vi "BattleShip.vi"() -> ()   [LabVIEW 2015]
uses:
  <vilib>/Utility/miscctls.llb/LVMouseTypeDef.ctl
  <vilib>/Utility/miscctls.llb/LVPoint32TypeDef.ctl
  <vilib>/Utility/miscctls.llb/LVPositionTypeDef.ctl
  <vilib>/picture/picture.llb/Draw True-Color Pixmap.vi
panel:
  out "appended path":path
  out "path":path
  out "BasePath":path
  in  "PlayMusic":i32
  out "HitIndex 4":u32
  out "HitIndex 3":u32
  out "Enum":T1(ring)
  out "TimeToChangeTurn":bool
  in  "First":bool
  in  "Counter":i32
  out "timed out 3":bool
  out "TimeToChangeTurn2 2":bool
  out "TimeToChangeTurn2":bool
  out "HitIndex 2":u32
  out "x .and. y? 4":bool
  out "x .and. y? 3":bool
  out "x .and. y? 2":bool
  out "x .and. y?":bool
  out "DataTemp":T2
  out "SendFormat":T2
  out "SendLocation":cluster{i32, i32}
  out "HitIndex":u32
  out "timed out 2":bool
  out "InputFromEnermy 2":T3
  out "timed out":bool
  out "InputFromEnermy":T3
  out "HitArray":picture[](array[picture])
  out "HitPicture":picture
  in  "MouseButtonDown":bool=TRUE
  out "Boolean":bool
  out "MouseLocation":T4
  out "Mouse Position":cluster{"X":i32, "Y":i32}
  in  "ClientFirst?":bool
  in  "URLReceive":string="dstp://localhost/dddd"
  in  "URLSend":string="dstp://localhost/wave"
  in  "BattleShipFace":bool[][](array[boolean])
  in  "BackGroundFace":bool[][](array[boolean])
  out "Mouse":T5
  out "InitArray":cluster{i32, i32}[](array[cluster])
  out "ShipFourArray":cluster{i32, i32}[][](array[cluster])
  out "ShipThreeArray":cluster{i32, i32}[][](array[cluster])
  out "ShipTwoArray":cluster{i32, i32}[][](array[cluster])
  out "ShipOneArray":cluster{i32, i32}[][](array[cluster])
  in  "ReadyButton":bool
  out "ShipMap":u32[][](array[numeric])
  out "ShipsNumber":i32[](array[numeric])
  in  "PictureButtonDown":bool
  out "ShipFourPixmap":u32[][](array[numeric]) format="%x"
  out "ShipThreePixmap":u32[][](array[numeric]) format="%x"
  out "ShipTwoPixmap":u32[][](array[numeric]) format="%x"
  out "ShipOnePixmap":u32[][](array[numeric]) format="%x"
  in  "Direction":i32
  out "PictureOut":picture
  in  "ShipChoose":i32
  out "BackGround":picture
  in  "ShipFour":bool
  in  "ShipThree":bool
  in  "ShipTwo":bool
  in  "ShipOne":bool
  in  "Array":bool[][](array[boolean])
  # "1.BattleShip的URLSend 要跟 BattleShip2的URLReceive 一樣\nBattleShip的 URLReceive 要跟 BattleShip2 的 URLSend 一樣\n，基本上用其中一個人的IP即可\nEX : BattleShip:\n            URLSend : dstp://140.113.89.154/wave \n            URLReceive : dstp://140.113.89.154/dddd\n         BattleShip2:\n            URLSend : dstp://140.113.89.154/dddd \n            URLReceive : dstp://140.113.89.154/wave\n\n\n2.一開始會先把船放到自己右邊的地圖上，然後每種船有固定的數量，按空白\n鍵可以轉船的方向，放完後，按Ready進入ReadyAndWait狀態，等BattleShip2\n的人也按Ready。如果連線成功，一方會進入MyTurn，另一邊會進入EnermyTurn\n，MyTurn的人可以用滑鼠按右邊地圖猜對面船的位子，如果猜中就可以繼續猜，\n沒中就要換邊，如果全部猜完，遊戲就會結束。\n\n3.連線後右邊是別人的地圖，左邊是自己的"
  # "遊戲狀態"
  # "Cruiser*4"
  # "Chaser*2"
  # "SubMarine*2"
  # "BattleShip*1"
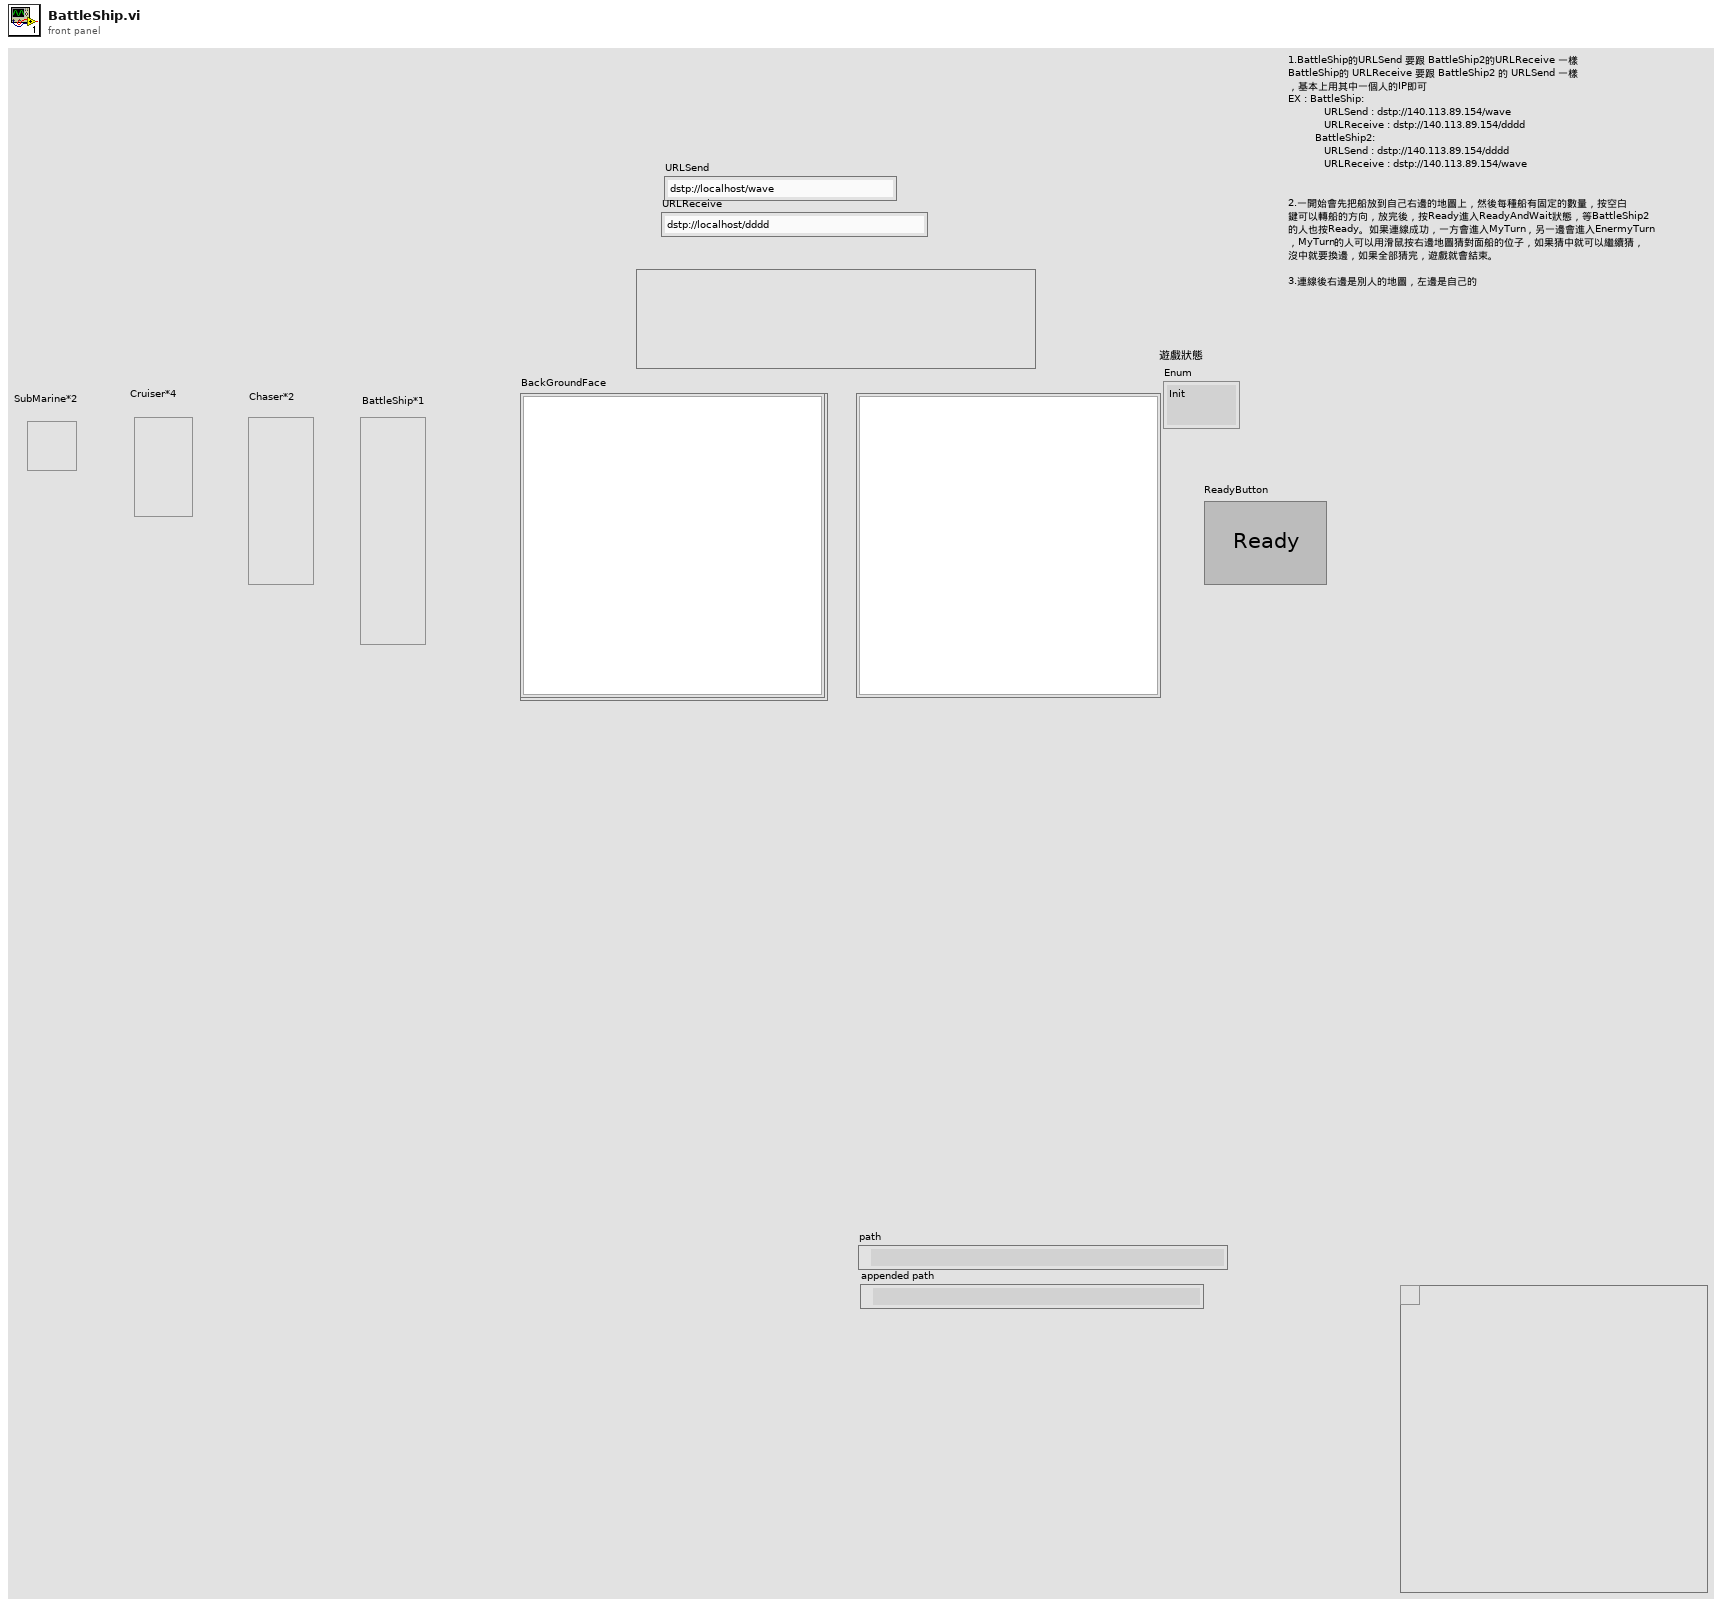
[diagram p1: front panel]
types:
  T1 = enum16{"Init", "Wait", "ReadyAndWait", "MyTurn", "EnermyTurn", "GameOver"}
  T2 = cluster{"HitIndex":u32, "SendLocation":cluster{i32, i32}}
  T3 = cluster{"BackGround":picture, "ShipMap":u32[][], "ShipOneArray":cluster{i32, i32}[][], "ShipTwoArray":cluster{i32, i32}[][], "ShipThreeArray":cluster{i32, i32}[][], "ShipFourArray":cluster{i32, i32}[][]}
  T4 = typedef "LVPoint32TypeDef.ctl" = cluster{"Horizontal":i32, "Vertical":i32}
  T5 = typedef "LVMouseTypeDef.ctl" = cluster{"Mouse Position":cluster{"X":i32, "Y":i32}, "Mouse Modifiers":cluster{"Button Down":bool, "Shift Mod":bool, "Menu Mod":bool, "Option Mod":bool}}
  T6 = enum16{"Init", "Wait", "ReadyAndWait", "MyTurn", "EnermyTurn"}
  T7 = cluster{"Button Down":bool, "Shift Mod":bool, "Menu Mod":bool, "Option Mod":bool}
  T8 = enum8{"Enabled", "Disabled", "Disabled and Grayed Out"}
  T9 = typedef "LVPositionTypeDef.ctl" = cluster{"Left":i32, "Top":i32}
  T10 = enum16{"Read", "Write", "ReadWrite", "BufferedRead", "BufferedReadWrite"}
  T11 = typedef "imagedata.ctl" = cluster{"image type":i32, "image depth":i32, "image":u8[], "mask":u8[], "colors":u32[], "Rectangle":cluster{"left":i16, "top":i16, "right":i16, "bottom":i16}}
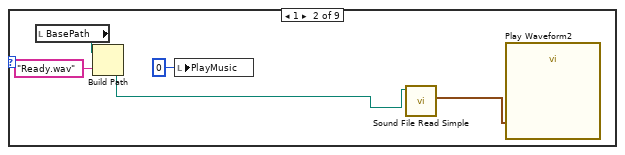
[diagram p3: hidden frame]
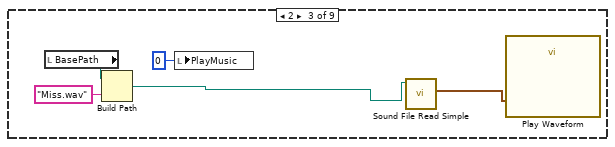
[diagram p4: hidden frame]
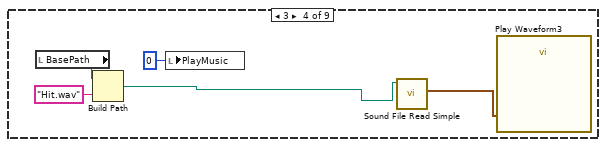
[diagram p5: hidden frame]
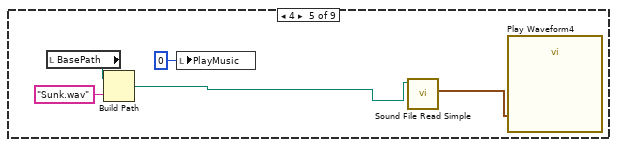
[diagram p6: hidden frame]
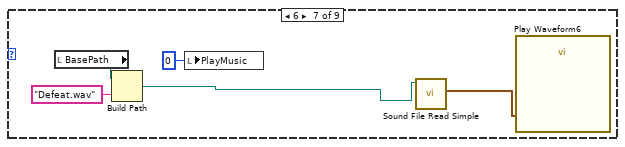
[diagram p7: hidden frame]
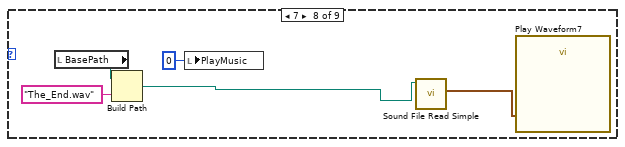
[diagram p8: hidden frame]
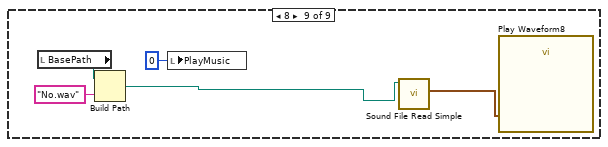
[diagram p9: hidden frame]
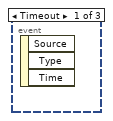
[diagram p10: hidden frame]
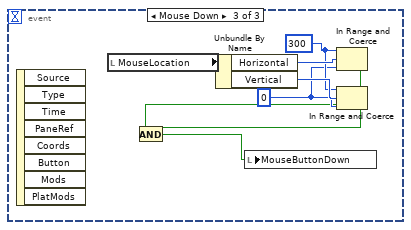
[diagram p11: hidden frame]
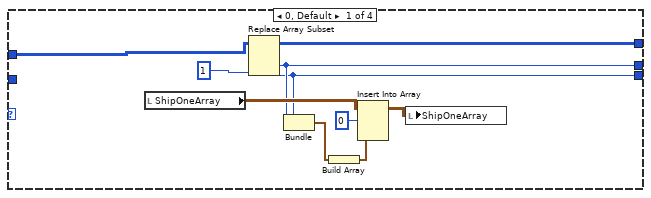
[diagram p13: hidden frame]
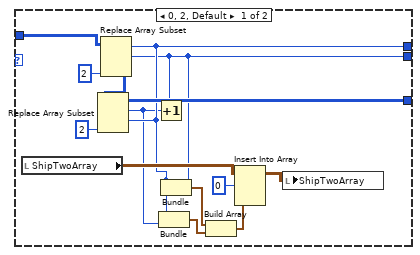
[diagram p14: hidden frame]
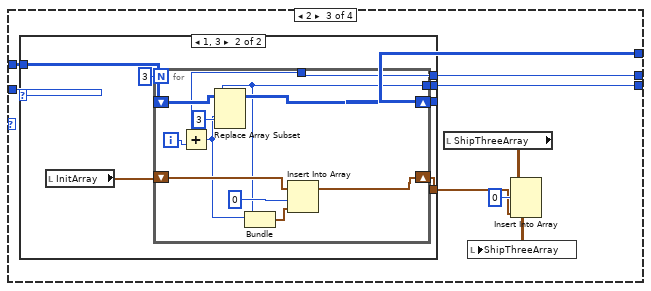
[diagram p15: hidden frame]
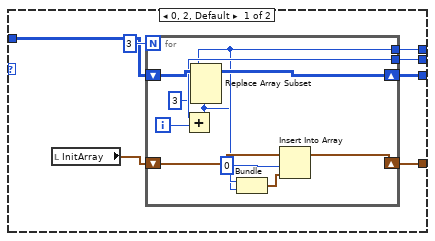
[diagram p16: hidden frame]
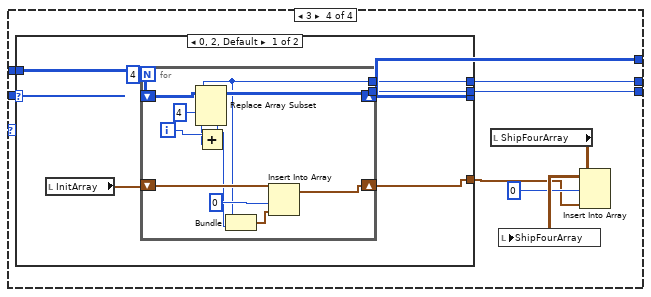
[diagram p17: hidden frame]
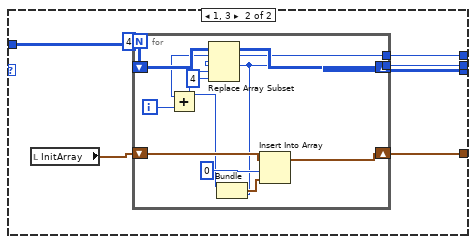
[diagram p18: hidden frame]
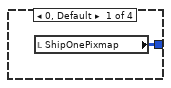
[diagram p19: hidden frame]
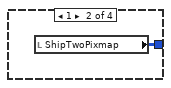
[diagram p20: hidden frame]
diagram:
  # "有五個State\n1.Init :\n           初始化必要的變數\n2.Wait:\n           畫製自己的地圖\n3.ReadyAndWait:\n           跟對方連線、傳資料\n4.MyTurn:\n           可以按右邊的地圖猜對方船的位子\n5.EnermyTurn:\n           對方的回合，被擊中的地方會畫上X\n6.GameOver:\n           遊戲結束"
  # "選定要放的音樂"
  # "在右邊的地圖上按滑鼠左鍵可以把選到的船印在圖上"
  # "把滑鼠移到右邊的地圖上時，會顯示應該會呈現的圖案"
  n1 = while {
    stop <- FALSE stop-if-true
    n2 = local read "Enum"() -> (w8:T1)
    n3 = Equal?(x=w8, y=T6."Wait") -> (x = y?=w7:bool)
    n4 = case shown="True" w7 {
      frame False {
      }
      frame True {
        w19 = 20 ("y")
        w25 = 20 ("y")
        n5 = local read "ShipChoose"() -> (w15:i32)
        n6 = case shown="3" w15 {
          tunnel: [w30 w31 w32 w33] -> w14
          frame 0, Default {
            n7 = local read "ShipOnePixmap"() -> (w30:u32[][])
          }
          frame 1 {
            n8 = local read "ShipTwoPixmap"() -> (w31:u32[][])
          }
          frame 2 {
            n9 = local read "ShipThreePixmap"() -> (w32:u32[][])
          }
          frame 3 {
            n10 = local read "ShipFourPixmap"() -> (w33:u32[][])
          }
        }
        n11 = property on="PictureOut" class="Pict"() -> ("Mouse"=w18:T5)  [unwired: 2 in, 2 out]
        n12 = local read "Direction"() -> (w17:i32)
        n13 = local read "BackGround"() -> (w28:picture)
        n14 = Unbundle By Name(w18) -> ("Mouse Position"=w29:cluster{"X":i32, "Y":i32}, "Mouse Modifiers"=w13:T7)
        "Mouse Position" <- w29
        n15 = case shown="3" w17 {
          tunnel: w14 -> [w34 w36 w40 w45]
          tunnel: [w34 w35 w37 w43] -> w16
          frame 0, Default {
          }
          frame 1 {
            n16 = Transpose 2D Array(2D array=w36) -> (transposed array=w35:u32[][])
          }
          frame 2 {
            n17 = Transpose 2D Array(2D array=w40) -> (transposed array=w39:u32[][])
            n18 = for {
              tunnel: w39 -> [w42] mode=indexing
              tunnel: [w41] -> w38 mode=indexing
              n19 = Reverse 1D Array(array=w42) -> (reversed array=w41:u32[])
            }
            n20 = Transpose 2D Array(2D array=w38) -> (transposed array=w37:u32[][])
          }
          frame 3 {
            n21 = Transpose 2D Array(2D array=w45) -> (transposed array=w44:u32[][])
            n22 = for {
              tunnel: w44 -> [w47] mode=indexing
              tunnel: [w46] -> w43 mode=indexing
              n23 = Reverse 1D Array(array=w47) -> (reversed array=w46:u32[])
            }
          }
        }
        n24 = Unbundle By Name(w13) -> ("Button Down"=w12:bool)
        n25 = Unbundle By Name(w29) -> ("X"=w27:i32, "Y"=w26:i32)
        n26 = Quotient & Remainder(x=w27, y=w25) -> (floor(x/y)=w21:i32)  [unwired: 1 out]
        n27 = Quotient & Remainder(x=w26, y=w25) -> (floor(x/y)=w22:i32)  [unwired: 1 out]
        n28 = local write "PictureButtonDown"(w12) -> ()
        n29 = Multiply(x=w21, y=w19) -> (x*y=w23:i32)
        n30 = Multiply(x=w19, y=w22) -> (x*y=w20:i32)
        n31 = Bundle(w23, w20) -> (w24:cluster{i32, i32})  [unwired: 1 in]
        n32 = call-poly <vilib>:"Draw Unflattened Pixmap.vi"("picture"=w28, "top left point(0, 0)"=w24, "data (RGB format)"=w16) -> ("new picture"=w11:picture)  [unwired: 6 in]
        n33 = local write "PictureOut"(w11) -> ()
      }
    }
  }
  n34 = while {
    stop <- FALSE stop-if-true
    n35 = local read "ShipsNumber"() -> (w52:i32[])
    n36 = local read "ShipChoose"() -> (w51:i32)
    n37 = local read "PictureButtonDown"() -> (w54:bool)
    n38 = Index Array(array=w52, index=w51) -> (element=w50:i32)
    n39 = Greater Than 0?(x=w50) -> (x > 0?=w49:bool)
    n40 = And(x=w54, y=w49) -> (x .and. y?=w53:bool)
    n41 = case shown="True" w53 {
      frame False {
      }
      frame True {
        w77 = 20 ("y")
        w73 = 20 ("y")
        n42 = local read "ShipsNumber"() -> (w63:i32[])
        n43 = local read "ShipChoose"() -> (w61:i32)
        n44 = case shown="3" w61 {
          tunnel: [w212 w213 w214 w215] -> w79
          frame 0, Default {
            n45 = local read "ShipOnePixmap"() -> (w212:u32[][])
          }
          frame 1 {
            n46 = local read "ShipTwoPixmap"() -> (w213:u32[][])
          }
          frame 2 {
            n47 = local read "ShipThreePixmap"() -> (w214:u32[][])
          }
          frame 3 {
            n48 = local read "ShipFourPixmap"() -> (w215:u32[][])
          }
        }
        n49 = property on="PictureOut" class="Pict"() -> ("Mouse"=w68:T5)  [unwired: 2 in, 2 out]
        n50 = local read "ShipMap"() -> (w60:u32[][])
        n51 = local read "Direction"() -> (w56:i32)
        n52 = Index Array(array=w63, index=w61) -> (element=w64:i32)
        n53 = Decrement(x=w64) -> (x-1=w66:i32)
        n54 = local read "BackGround"() -> (w70:picture)
        n55 = Replace Array Subset(array=w63, new element=w66, index=w61) -> (w65:i32[])
        n56 = Unbundle By Name(w68) -> ("Mouse Position"=w69:cluster{"X":i32, "Y":i32})
        n57 = case shown="3" w56 {
          tunnel: w79 -> [w216 w218 w222 w227]
          tunnel: [w216 w217 w219 w225] -> w78
          frame 0, Default {
          }
          frame 1 {
            n58 = Transpose 2D Array(2D array=w218) -> (transposed array=w217:u32[][])
          }
          frame 2 {
            n59 = Transpose 2D Array(2D array=w222) -> (transposed array=w221:u32[][])
            n60 = for {
              tunnel: w221 -> [w224] mode=indexing
              tunnel: [w223] -> w220 mode=indexing
              n61 = Reverse 1D Array(array=w224) -> (reversed array=w223:u32[])
            }
            n62 = Transpose 2D Array(2D array=w220) -> (transposed array=w219:u32[][])
          }
          frame 3 {
            n63 = Transpose 2D Array(2D array=w227) -> (transposed array=w226:u32[][])
            n64 = for {
              tunnel: w226 -> [w229] mode=indexing
              tunnel: [w228] -> w225 mode=indexing
              n65 = Reverse 1D Array(array=w229) -> (reversed array=w228:u32[])
            }
          }
        }
        n66 = local write "ShipsNumber"(w65) -> ()
        n67 = Unbundle By Name(w69) -> ("X"=w71:i32, "Y"=w72:i32)
        n68 = Quotient & Remainder(x=w71, y=w73) -> (floor(x/y)=w59:i32)  [unwired: 1 out]
        n69 = Quotient & Remainder(x=w72, y=w73) -> (floor(x/y)=w58:i32)  [unwired: 1 out]
        n70 = case shown="1" w61 {
          tunnel: w60 -> [w89 w93 w129 w174]
          tunnel: w59 -> [w84 w91 w127 w171]
          tunnel: w58 -> [w83 w92 w128 w172]
          tunnel: [w87 w90 w126 w173] -> w57
          tunnel: w56 -> [_ w94 w130 w175]
          frame 0, Default {
            n71 = local read "ShipOneArray"() -> (w85:cluster{i32, i32}[][])
            n72 = Replace Array Subset(array=w89, new element=u32 1 ("new element/subarray"), index (row)=w83, index (col)=w84) -> (w87:u32[][])
            n73 = Bundle(w84, w83) -> (w82:cluster{i32, i32})  [unwired: 1 in]
            n74 = Build Array(w82) -> (w81:cluster{i32, i32}[])
            n75 = Insert Into Array(array=w85, index (row)=0 ("index"), new element=w81) -> (w80:cluster{i32, i32}[][])  [unwired: 1 in]
            n76 = local write "ShipOneArray"(w80) -> ()
          }
          frame 1 {
            n77 = case shown="1, 3" w94 {
              tunnel: w93 -> [w108 w121]
              tunnel: w92 -> [w96 w109]
              tunnel: w91 -> [w97 w110]
              tunnel: [w104 w118] -> w90
              frame 0, 2, Default {
                n78 = local read "ShipTwoArray"() -> (w102:cluster{i32, i32}[][])
                n79 = Replace Array Subset(array=w108, new element=u32 2 ("new element/subarray"), index (row)=w96, index (col)=w97) -> (w105:u32[][])
                n80 = Increment(x=w96) -> (x+1=w95:i32)
                n81 = Replace Array Subset(array=w105, new element=u32 2 ("new element/subarray"), index (row)=w95, index (col)=w97) -> (w104:u32[][])
                n82 = Bundle(w97, w95) -> (w98:cluster{i32, i32})  [unwired: 1 in]
                n83 = Bundle(w97, w96) -> (w101:cluster{i32, i32})  [unwired: 1 in]
                n84 = Build Array(w101, w98) -> (w100:cluster{i32, i32}[])
                n85 = Insert Into Array(array=w102, index (row)=0 ("index"), new element=w100) -> (w99:cluster{i32, i32}[][])  [unwired: 1 in]
                n86 = local write "ShipTwoArray"(w99) -> ()
              }
              frame 1, 3 {
                w119 = u32 2 ("new element/subarray")
                n87 = local read "ShipTwoArray"() -> (w116:cluster{i32, i32}[][])
                n88 = Replace Array Subset(array=w121, new element=w119, index (row)=w109, index (col)=w110) -> (w120:u32[][])
                n89 = Increment(x=w110) -> (x+1=w111:i32)
                n90 = Replace Array Subset(array=w120, new element=w119, index (row)=w109, index (col)=w111) -> (w118:u32[][])
                n91 = Bundle(w111, w109) -> (w112:cluster{i32, i32})  [unwired: 1 in]
                n92 = Bundle(w110, w109) -> (w115:cluster{i32, i32})  [unwired: 1 in]
                n93 = Build Array(w115, w112) -> (w114:cluster{i32, i32}[])
                n94 = Insert Into Array(array=w116, index (row)=0 ("index"), new element=w114) -> (w113:cluster{i32, i32}[][])  [unwired: 1 in]
                n95 = local write "ShipTwoArray"(w113) -> ()
              }
            }
          }
          frame 2 {
            n96 = case shown="1, 3" w130 {
              tunnel: w129 -> [w136 w154]
              tunnel: w128 -> [w135 w152]
              tunnel: w127 -> [w134 w153]
              tunnel: [w133 w151] -> w126
              tunnel: [w131 w149] -> w123
              frame 0, 2, Default {
                n97 = local read "InitArray"() -> (w132:cluster{i32, i32}[])
                n98 = for {
                  N: 3 -> [_]
                  shift-right: [w147] -> w133
                  shift-left: w136 -> [w148]
                  tunnel: w135 -> [w145]
                  tunnel: w134 -> [w141]
                  shift-right: [w138] -> w131
                  shift-left: w132 -> [w143]
                  i -> [w146]
                  n99 = Add(x=w145, y=w146) -> (x+y=w140:i32)
                  n100 = Replace Array Subset(array=w148, new element=u32 3 ("new element/subarray"), index (row)=w140, index (col)=w141) -> (w147:u32[][])
                  n101 = Bundle(w141, w140) -> (w139:cluster{i32, i32})  [unwired: 1 in]
                  n102 = Insert Into Array(array=w143, index=0, new element=w139) -> (w138:cluster{i32, i32}[])
                }
              }
              frame 1, 3 {
                n103 = local read "InitArray"() -> (w150:cluster{i32, i32}[])
                n104 = for {
                  N: 3 -> [_]
                  shift-right: [w165] -> w151
                  shift-left: w154 -> [w166]
                  tunnel: w153 -> [w163]
                  tunnel: w152 -> [w156]
                  shift-right: [w158] -> w149
                  shift-left: w150 -> [w159]
                  i -> [w164]
                  n105 = Add(x=w163, y=w164) -> (x+y=w157:i32)
                  n106 = Replace Array Subset(array=w166, new element=u32 3 ("new element/subarray"), index (row)=w156, index (col)=w157) -> (w165:u32[][])
                  n107 = Bundle(w157, w156) -> (w160:cluster{i32, i32})  [unwired: 1 in]
                  n108 = Insert Into Array(array=w159, index=0, new element=w160) -> (w158:cluster{i32, i32}[])
                }
              }
            }
            n109 = local read "ShipThreeArray"() -> (w125:cluster{i32, i32}[][])
            n110 = Insert Into Array(array=w125, index (row)=0, new element=w123) -> (w122:cluster{i32, i32}[][])  [unwired: 1 in]
            n111 = local write "ShipThreeArray"(w122) -> ()
          }
          frame 3 {
            n112 = case shown="0, 2, Default" w175 {
              tunnel: w174 -> [w182 w199]
              tunnel: [w181 w196] -> w173
              tunnel: w172 -> [w179 w197]
              tunnel: w171 -> [w178 w198]
              tunnel: [w176 w194] -> w167
              frame 0, 2, Default {
                n113 = local read "InitArray"() -> (w177:cluster{i32, i32}[])
                n114 = for {
                  N: 4 -> [_]
                  shift-right: [w192] -> w181
                  shift-left: w182 -> [w193]
                  tunnel: w179 -> [w190]
                  tunnel: w178 -> [w183]
                  shift-right: [w185] -> w176
                  shift-left: w177 -> [w186]
                  i -> [w191]
                  n115 = Add(x=w191, y=w190) -> (x+y=w184:i32)
                  n116 = Replace Array Subset(array=w193, new element=u32 4 ("new element/subarray"), index (row)=w184, index (col)=w183) -> (w192:u32[][])
                  n117 = Bundle(w183, w184) -> (w187:cluster{i32, i32})  [unwired: 1 in]
                  n118 = Insert Into Array(array=w186, index=0, new element=w187) -> (w185:cluster{i32, i32}[])
                }
              }
              frame 1, 3 {
                n119 = local read "InitArray"() -> (w195:cluster{i32, i32}[])
                n120 = for {
                  N: 4 -> [_]
                  shift-right: [w210] -> w196
                  shift-left: w199 -> [w211]
                  tunnel: w198 -> [w203]
                  tunnel: w197 -> [w201]
                  shift-right: [w204] -> w194
                  shift-left: w195 -> [w205]
                  i -> [w209]
                  n121 = Add(x=w203, y=w209) -> (x+y=w202:i32)
                  n122 = Replace Array Subset(array=w211, new element=u32 4 ("new element/subarray"), index (row)=w201, index (col)=w202) -> (w210:u32[][])
                  n123 = Bundle(w202, w201) -> (w206:cluster{i32, i32})  [unwired: 1 in]
                  n124 = Insert Into Array(array=w205, index=0, new element=w206) -> (w204:cluster{i32, i32}[])
                }
              }
            }
            n125 = local read "ShipFourArray"() -> (w169:cluster{i32, i32}[][])
            n126 = Insert Into Array(array=w169, index (row)=0 ("index"), new element=w167) -> (w170:cluster{i32, i32}[][])  [unwired: 1 in]
            n127 = local write "ShipFourArray"(w170) -> ()
          }
        }
        n128 = Multiply(x=w59, y=w77) -> (x*y=w75:i32)
        n129 = Multiply(x=w77, y=w58) -> (x*y=w76:i32)
        n130 = Bundle(w75, w76) -> (w74:cluster{i32, i32})  [unwired: 1 in]
        n131 = call-poly <vilib>:"Draw Unflattened Pixmap.vi"("picture"=w70, "top left point(0, 0)"=w74, "data (RGB format)"=w78) -> ("new picture"=w67:picture)  [unwired: 6 in]
        n132 = local write "ShipMap"(w57) -> ()
        n133 = local write "BackGround"(w67) -> ()
        n134 = Wait Until Next ms Multiple(millisecond multiple=u32 1500) -> ()  [unwired: 1 out]
      }
    }
    n135 = property on="PictureOut" class="Pict"() -> ("Mouse"=→"Mouse":T5)  [unwired: 2 in, 2 out]
  }
  n136 = while {
    shift-right: [w231] -> _
    shift-left: T1."Init" -> [w230]
    stop <- FALSE stop-if-true
    n137 = case shown="\"Wait\"" w230 {
      tunnel: [enum16{"Init", "Wait"}."Wait" enum16{"Init", "Wait"}."Wait" w345 w391 w510 w751 T1."GameOver"] -> w231
      frame "Init" {
        w285 = FALSE
        w300 = 15
        w303 = 15
        n138 = local write "ShipChoose"(0 ("ShipChoose")) -> ()
        n139 = Initialize Array(cluster{i32, i32} {0, 0}, 0 ("dimension size"), 0 ("dimension size")) -> (→"ShipOneArray" →"ShipTwoArray" →"ShipThreeArray" →"ShipFourArray":cluster{i32, i32}[][])
        n140 = local write "PlayMusic"(0 ("PlayMusic")) -> ()
        n141 = local write "Direction"(0 ("Direction")) -> ()
        n142 = Initialize Array(u32 0 ("element"), 15 ("dimension size"), 15 ("dimension size")) -> (→"ShipMap":u32[][])
        n143 = Build Array(2, 4, 2, 1) -> (→"ShipsNumber":i32[])
        n144 = local read "BasePath"() -> (w276:path)
        n145 = local read "BasePath"() -> (w272:path)
        n146 = Build Path(base path=w276, name or relative path="ShipTwo.png") -> (appended path=w277:path)
        n147 = call <vilib>:"Read PNG File.vi"("path to PNG file"=w277) -> ("image data"=w341:T11)  [unwired: 8 in, 2 out]
        n148 = call <vilib>:"Unflatten Pixmap.vi"("image data"=w341) -> ("24-bit pixmap"=→"ShipTwoPixmap":u32[][])  [unwired: 4 in, 6 out]
        n149 = Build Path(base path=w276, name or relative path="BackGroundWhite.png") -> (appended path=w281:path)
        n150 = call <vilib>:"Read PNG File.vi"("path to PNG file"=w281) -> ("image data"=w337:T11)  [unwired: 8 in, 2 out]
        n151 = call <vilib>:"Unflatten Pixmap.vi"("image data"=w337) -> ("24-bit pixmap"=w336:u32[][])  [unwired: 4 in, 6 out]
        n152 = call-poly <vilib>:"Draw Unflattened Pixmap.vi"("data (RGB format)"=w336) -> ("new picture"=w335:picture)  [unwired: 8 in]
        n153 = local write "BackGround"(w335) -> ()
        n154 = Build Path(base path=w272, name or relative path="ShipThree.png") -> (appended path=w271:path)
        n155 = call <vilib>:"Read PNG File.vi"("path to PNG file"=w271) -> ("image data"=w340:T11)  [unwired: 8 in, 2 out]
        n156 = call <vilib>:"Unflatten Pixmap.vi"("image data"=w340) -> ("24-bit pixmap"=→"ShipThreePixmap":u32[][])  [unwired: 4 in, 6 out]
        n157 = Build Path(base path=w276, name or relative path="ShipOne.png") -> (appended path=w278:path)
        n158 = call <vilib>:"Read PNG File.vi"("path to PNG file"=w278) -> ("image data"=w342:T11)  [unwired: 8 in, 2 out]
        n159 = call <vilib>:"Unflatten Pixmap.vi"("image data"=w342) -> ("24-bit pixmap"=→"ShipOnePixmap":u32[][])  [unwired: 4 in, 6 out]
        n160 = Build Path(base path=w272, name or relative path="ShipFour.png") -> (appended path=w270:path)
        n161 = call <vilib>:"Read PNG File.vi"("path to PNG file"=w270) -> ("image data"=w339:T11)  [unwired: 8 in, 2 out]
        n162 = call <vilib>:"Unflatten Pixmap.vi"("image data"=w339) -> ("24-bit pixmap"=→"ShipFourPixmap":u32[][])  [unwired: 4 in, 6 out]
        n163 = local read "BasePath"() -> (w260:path)
        n164 = local read "BasePath"() -> (w263:path)
        n165 = local read "BasePath"() -> (w268:path)
        n166 = local read "BasePath"() -> (w267:path)
        n167 = local read "BasePath"() -> (w264:path)
        n168 = Build Path(base path=w260, name or relative path="HitBattleship.png") -> (appended path=w255:path)
        n169 = Build Path(base path=w263, name or relative path="HitChaser.png") -> (appended path=w256:path)
        n170 = Build Path(base path=w268, name or relative path="TextBackGround.png") -> (appended path=w259:path)
        n171 = Build Path(base path=w267, name or relative path="HitSubMarine.png") -> (appended path=w258:path)
        n172 = Build Path(base path=w264, name or relative path="HitCruiser.png") -> (appended path=w257:path)
        n173 = property on="BackGroundFace" class="Arr (strict)"("DisabledEnum"=T8."Disabled" ("Disabled")) -> ()  [unwired: 2 in, 2 out]
        n174 = local write "ClientFirst?"(TRUE ("ClientFirst?")) -> ()
        n175 = local write "HitIndex 2"(u32 0 ("HitIndex 2")) -> ()
        n176 = local write "HitIndex"(u32 0 ("HitIndex 2")) -> ()
        n177 = local read "BasePath"() -> (w244:path)
        n178 = local read "BasePath"() -> (w245:path)
        n179 = local read "BasePath"() -> (w253:path)
        n180 = local read "BasePath"() -> (w252:path)
        n181 = local read "BasePath"() -> (w248:path)
        n182 = local read "BasePath"() -> (w249:path)
        n183 = Build Path(base path=w244, name or relative path="SunkBattleShip.png") -> (appended path=w239:path)
        n184 = Build Path(base path=w245, name or relative path="Win.png") -> (appended path=w238:path)
        n185 = Build Path(base path=w253, name or relative path="SunkSubmarine.png") -> (appended path=w242:path)
        n186 = Build Path(base path=w252, name or relative path="SunkCruiser.png") -> (appended path=w241:path)
        n187 = Build Path(base path=w248, name or relative path="Lose.png") -> (appended path=w237:path)
        "appended path" <- w237
        n188 = Build Path(base path=w249, name or relative path="SunkChaser.png") -> (appended path=w240:path)
        n189 = Initialize Array(FALSE, w303, w303) -> (w298:bool[][])
        n190 = Initialize Array(FALSE, w300, w300) -> (w299:bool[][])
        n191 = local write "BattleShipFace"(w299) -> ()
        n192 = local write "BackGroundFace"(w298) -> ()
        n193 = property on="BattleShipFace" class="Arr (strict)"("Position"=T9 {"Left"=1000, "Top"=1000}) -> ()  [unwired: 2 in, 2 out]
        n194 = local write "MouseButtonDown"(FALSE ("MouseButtonDown")) -> ()
        n195 = local write "TimeToChangeTurn"(w285) -> ()
        n196 = local write "TimeToChangeTurn2"(w285) -> ()
        n197 = property on="Boolean" class="Bool (strict)"("Position"=T9 {"Left"=1000, "Top"=1000}) -> ()  [unwired: 2 in, 2 out]
        n198 = call <vilib>:"Read PNG File.vi"("path to PNG file"=w237) -> ("image data"=w289:T11)  [unwired: 8 in, 2 out]
        n199 = call <vilib>:"Read PNG File.vi"("path to PNG file"=w238) -> ("image data"=w288:T11)  [unwired: 8 in, 2 out]
        n200 = call <vilib>:"Read PNG File.vi"("path to PNG file"=w255) -> ("image data"=w311:T11)  [unwired: 8 in, 2 out]
        n201 = call <vilib>:"Read PNG File.vi"("path to PNG file"=w241) -> ("image data"=w296:T11)  [unwired: 8 in, 2 out]
        n202 = call <vilib>:"Read PNG File.vi"("path to PNG file"=w258) -> ("image data"=w314:T11)  [unwired: 8 in, 2 out]
        n203 = call <vilib>:"Read PNG File.vi"("path to PNG file"=w239) -> ("image data"=w294:T11)  [unwired: 8 in, 2 out]
        n204 = call <vilib>:"Read PNG File.vi"("path to PNG file"=w242) -> ("image data"=w297:T11)  [unwired: 8 in, 2 out]
        n205 = call <vilib>:"Read PNG File.vi"("path to PNG file"=w240) -> ("image data"=w295:T11)  [unwired: 8 in, 2 out]
        n206 = call <vilib>:"Read PNG File.vi"("path to PNG file"=w257) -> ("image data"=w313:T11)  [unwired: 8 in, 2 out]
        n207 = call <vilib>:"Read PNG File.vi"("path to PNG file"=w256) -> ("image data"=w312:T11)  [unwired: 8 in, 2 out]
        n208 = call <vilib>:"Read PNG File.vi"("path to PNG file"=w259) -> ("image data"=w310:T11)  [unwired: 8 in, 2 out]
        n209 = call <vilib>:"Draw Flattened Pixmap.vi"("image data"=w289) -> ("new picture"=w286:picture)  [unwired: 8 in]
        n210 = call <vilib>:"Draw Flattened Pixmap.vi"("image data"=w288) -> ("new picture"=w287:picture)  [unwired: 8 in]
        n211 = call <vilib>:"Draw Flattened Pixmap.vi"("image data"=w311) -> ("new picture"=w305:picture)  [unwired: 8 in]
        n212 = call <vilib>:"Draw Flattened Pixmap.vi"("image data"=w296) -> ("new picture"=w292:picture)  [unwired: 8 in]
        n213 = call <vilib>:"Draw Flattened Pixmap.vi"("image data"=w314) -> ("new picture"=w308:picture)  [unwired: 8 in]
        n214 = call <vilib>:"Draw Flattened Pixmap.vi"("image data"=w294) -> ("new picture"=w290:picture)  [unwired: 8 in]
        n215 = call <vilib>:"Draw Flattened Pixmap.vi"("image data"=w297) -> ("new picture"=w293:picture)  [unwired: 8 in]
        n216 = call <vilib>:"Draw Flattened Pixmap.vi"("image data"=w295) -> ("new picture"=w291:picture)  [unwired: 8 in]
        n217 = call <vilib>:"Draw Flattened Pixmap.vi"("image data"=w313) -> ("new picture"=w307:picture)  [unwired: 8 in]
        n218 = call <vilib>:"Draw Flattened Pixmap.vi"("image data"=w312) -> ("new picture"=w306:picture)  [unwired: 8 in]
        n219 = call <vilib>:"Draw Flattened Pixmap.vi"("image data"=w310) -> ("new picture"=w309:picture)  [unwired: 8 in]
        n220 = local write "First"(TRUE ("First")) -> ()
        n221 = Build Array(w309, w308, w307, w306, w305, w293, w292, w291, w290, w287, w286) -> (→"HitArray":picture[])
      }
      frame Default {
      }
      frame "Wait" {
        n222 = event shown="[6] \"ReadyButton\": Mouse Down" {
          selector: _ -> [_ _ _ _ _ _ _]
          dyn-events: _ -> [_ _ _ _ _ _ _]
          timeout: _ -> [_ _ _ _ _ _ _]
          tunnel: [_ enum16{"Init", "Wait", "ReadyAndWait"}."Wait" enum16{"Init", "Wait", "ReadyAndWait"}."Wait" enum16{"Init", "Wait", "ReadyAndWait"}."Wait" enum16{"Init", "Wait", "ReadyAndWait"}."Wait" enum16{"Init", "Wait", "ReadyAndWait"}."Wait" w381] -> w345
          event Timeout {
            n223 = event-data() -> ()  [unwired: 1 in, 3 out]
          }
          event "ShipOne": Mouse Down {
            w349 = 0 ("ShipChoose")
            n224 = event-data() -> ()  [unwired: 1 in, 8 out]
            n225 = local read "ShipsNumber"() -> (w352:i32[])
            n226 = Index Array(array=w352, index=w349) -> (element=w351:i32)
            n227 = local read "ShipChoose"() -> (w347:i32)
            n228 = Greater Than 0?(x=w351) -> (x > 0?=w350:bool)
            n229 = Select(t=w349, s=w350, f=w347) -> (s? t:f=w348:i32)
            n230 = local write "ShipChoose"(w348) -> ()
          }
          event "ShipTwo": Mouse Down {
            w356 = 1 ("ShipChoose")
            n231 = event-data() -> ()  [unwired: 1 in, 8 out]
            n232 = local read "ShipsNumber"() -> (w359:i32[])
            n233 = Index Array(array=w359, index=w356) -> (element=w358:i32)
            n234 = local read "ShipChoose"() -> (w354:i32)
            n235 = Greater Than 0?(x=w358) -> (x > 0?=w357:bool)
            n236 = Select(t=w356, s=w357, f=w354) -> (s? t:f=w355:i32)
            n237 = local write "ShipChoose"(w355) -> ()
          }
          event "ShipThree": Mouse Down {
            w365 = 2 ("ShipChoose")
            n238 = event-data() -> ()  [unwired: 1 in, 8 out]
            n239 = local read "ShipsNumber"() -> (w364:i32[])
            n240 = Index Array(array=w364, index=w365) -> (element=w363:i32)
            n241 = local read "ShipChoose"() -> (w366:i32)
            n242 = Greater Than 0?(x=w363) -> (x > 0?=w362:bool)
            n243 = Select(t=w365, s=w362, f=w366) -> (s? t:f=w361:i32)
            n244 = local write "ShipChoose"(w361) -> ()
          }
          event "ShipFour": Mouse Down {
            w370 = 3 ("ShipChoose")
            n245 = event-data() -> ()  [unwired: 1 in, 8 out]
            n246 = local read "ShipsNumber"() -> (w373:i32[])
            n247 = Index Array(array=w373, index=w370) -> (element=w372:i32)
            n248 = local read "ShipChoose"() -> (w368:i32)
            n249 = Greater Than 0?(x=w372) -> (x > 0?=w371:bool)
            n250 = Select(t=w370, s=w371, f=w368) -> (s? t:f=w369:i32)
            n251 = local write "ShipChoose"(w369) -> ()
          }
          event Key Down {
            n252 = event-data() -> ("ScanCode"=w375:i16)  [unwired: 1 in, 9 out]
            n253 = case shown="57" w375 {
              frame 0, Default {
              }
              frame 57 {
                n254 = local read "Direction"() -> (w379:i32)
                n255 = Increment(x=w379) -> (x+1=w378:i32)
                n256 = Quotient & Remainder(x=w378, y=4) -> (x-y*floor(x/y)=w376:i32)  [unwired: 1 out]
                n257 = local write "Direction"(w376) -> ()
              }
            }
          }
          event "ReadyButton": Mouse Down {
            n258 = event-data() -> ()  [unwired: 1 in, 8 out]
            n259 = local read "ShipsNumber"() -> (w385:i32[])
            n260 = for {
              shift-right: [w387] -> w384
              shift-left: TRUE -> [w388]
              tunnel: w385 -> [w390] mode=indexing
              n261 = Equal To 0?(x=w390) -> (x = 0?=w389:bool)
              n262 = And(x=w389, y=w388) -> (x .and. y?=w387:bool)
            }
            n263 = local write "PlayMusic"(1 ("PlayMusic")) -> ()
            n264 = Select(t=enum16{"Init", "Wait", "ReadyAndWait"}."ReadyAndWait", s=w384, f=enum16{"Init", "Wait", "ReadyAndWait"}."ReadyAndWait") -> (s? t:f=w381:enum16{"Init", "Wait", "ReadyAndWait"})
          }
        }
      }
      frame "ReadyAndWait" {
        n265 = flat-sequence {
          frame #0 {
            n266 = property on="PictureOut" class="Pict"() -> ("Position"=w399:T9)  [unwired: 2 in, 2 out]
            n267 = Unbundle By Name(w399) -> ("Left"=w400:i32, "Top"=w396:i32)
            n268 = Decrement(x=w400) -> (x-1=w397:i32)
            n269 = Decrement(x=w396) -> (x-1=w395:i32)
            n270 = Bundle(cluster=w399, "Left"=w397, "Top"=w395) -> (w398:T9)
            n271 = property on="BattleShipFace" class="Arr (strict)"("Position"=w398) -> ()  [unwired: 2 in, 2 out]
          }
          frame #1 {
            n272 = for {
              N: 15 -> [_]
              i -> [w405]
              n273 = Initialize Array(TRUE, 15 ("dimension size")) -> (w404:bool[])
              n274 = local read "BattleShipFace"() -> (w403:bool[][])
              n275 = Replace Array Subset(array=w403, new element=w404, index (row)=w405) -> (w402:bool[][])  [unwired: 1 in]
              n276 = Wait Until Next ms Multiple(millisecond multiple=u32 100) -> ()  [unwired: 1 out]
              n277 = local write "BattleShipFace"(w402) -> ()
            }
          }
          frame #2 {
            n278 = flat-sequence {
              frame #0 {
                n279 = local read "ClientFirst?"() -> (w409:bool)
                n280 = case shown="False" w409 {
                  frame False {
                    n281 = flat-sequence {
                      frame #0 {
                        n282 = local read "URLReceive"() -> (w412:string)
                        n283 = DataSocket Open(10:T10."Read" ("mode"), 11:w412) -> (3:w410:refnum<k13>)  [unwired: 2 in, 1 out]
                        n284 = while {
                          tunnel: w410 -> [w417]
                          stop <- w413 stop-if-true
                          n285 = DataSocket Read(10:"", 11:w417) -> (2:w415:string)  [unwired: 3 in, 6 out]
                          n286 = Equal?(x=w415, y="OK") -> (x = y?=w413:bool)
                        }
                      }
                      frame #1 {
                        n287 = local read "URLSend"() -> (w420:string)
                        n288 = DataSocket Open(10:T10."Write" ("mode"), 11:w420) -> (3:w418:refnum<k13>)  [unwired: 2 in, 1 out]
                        n289 = DataSocket Write(10:"ACK", 11:w418) -> ()  [unwired: 2 in, 3 out]
                      }
                    }
                  }
                  frame True {
                    n290 = flat-sequence {
                      tunnel: [w424] -> w423
                      tunnel: [w424] -> w422
                      tunnel: w423 -> [_]
                      tunnel: w422 -> [_]
                      frame #0 {
                        n291 = local read "URLSend"() -> (w427:string)
                        n292 = DataSocket Open(10:T10."Write" ("mode"), 11:w427) -> (3:w424:refnum<k13>)  [unwired: 2 in, 1 out]
                        n293 = DataSocket Write(10:"OK", 11:w424) -> ()  [unwired: 2 in, 3 out]
                      }
                      frame #1 {
                        n294 = local read "URLReceive"() -> (w429:string)
                        n295 = DataSocket Open(10:T10."Read" ("mode"), 11:w429) -> (3:w428:refnum<k13>)  [unwired: 2 in, 1 out]
                        n296 = while {
                          tunnel: w428 -> [w431]
                          stop <- w433 stop-if-true
                          w432 = "ACK"
                          n297 = DataSocket Read(10:w432, 11:w431) -> (2:w434:string)  [unwired: 3 in, 6 out]
                          n298 = Equal?(x=w434, y=w432) -> (x = y?=w433:bool)
                        }
                      }
                    }
                  }
                }
              }
              frame #1 {
                n299 = local read "ClientFirst?"() -> (w435:bool)
                n300 = case shown="False" w435 {
                  frame False {
                    n301 = local read "ShipFourArray"() -> (w442:cluster{i32, i32}[][])
                    n302 = local read "ShipTwoArray"() -> (w444:cluster{i32, i32}[][])
                    n303 = local read "ShipOneArray"() -> (w445:cluster{i32, i32}[][])
                    n304 = local read "ShipThreeArray"() -> (w443:cluster{i32, i32}[][])
                    n305 = local read "URLReceive"() -> (w438:string)
                    n306 = local read "BackGround"() -> (w447:picture)
                    n307 = local read "ShipMap"() -> (w446:u32[][])
                    n308 = DataSocket Open(10:T10."Read" ("mode"), 11:w438) -> (3:w436:refnum<k13>)  [unwired: 2 in, 1 out]
                    n309 = DataSocket Read(11:w436) -> (3:w437:refnum<k13>)  [unwired: 4 in, 6 out]
                    n310 = Bundle("BackGround"=w447, "ShipMap"=w446, "ShipOneArray"=w445, "ShipTwoArray"=w444, "ShipThreeArray"=w443, "ShipFourArray"=w442) -> (w441:T3)  [unwired: 1 in]
                    n311 = while {
                      tunnel: [w452] -> w440
                      tunnel: w441 -> [w449]
                      tunnel: w437 -> [w448]
                      stop <- w453 stop-if-true
                      n312 = DataSocket Read(9:1000 ("ms timeout (10000)"), 10:w449, 11:w448) -> (1:w450:bool, 2:w452:T3)  [unwired: 2 in, 5 out]
                      "timed out" <- w450
                      n313 = Not(x=w450) -> (.not. x?=w453:bool)
                    }
                    "InputFromEnermy" <- w440
                  }
                  frame True {
                    n314 = local read "URLSend"() -> (w456:string)
                    n315 = local read "ShipFourArray"() -> (w458:cluster{i32, i32}[][])
                    n316 = local read "ShipTwoArray"() -> (w460:cluster{i32, i32}[][])
                    n317 = local read "ShipOneArray"() -> (w461:cluster{i32, i32}[][])
                    n318 = local read "ShipThreeArray"() -> (w459:cluster{i32, i32}[][])
                    n319 = local read "BackGround"() -> (w463:picture)
                    n320 = local read "ShipMap"() -> (w462:u32[][])
                    n321 = DataSocket Open(10:T10."Write" ("mode"), 11:w456) -> (3:w454:refnum<k13>)  [unwired: 2 in, 1 out]
                    n322 = Bundle("BackGround"=w463, "ShipMap"=w462, "ShipOneArray"=w461, "ShipTwoArray"=w460, "ShipThreeArray"=w459, "ShipFourArray"=w458) -> (w457:T3)  [unwired: 1 in]
                    n323 = DataSocket Write(10:w457, 11:w454) -> ()  [unwired: 2 in, 3 out]
                  }
                }
              }
              frame #2 {
                n324 = local read "ClientFirst?"() -> (w465:bool)
                n325 = Not(x=w465) -> (.not. x?=w464:bool)
                n326 = case shown="False" w464 {
                  frame False {
                    n327 = local read "URLReceive"() -> (w469:string)
                    n328 = local read "ShipFourArray"() -> (w472:cluster{i32, i32}[][])
                    n329 = local read "ShipTwoArray"() -> (w474:cluster{i32, i32}[][])
                    n330 = local read "ShipOneArray"() -> (w475:cluster{i32, i32}[][])
                    n331 = local read "ShipThreeArray"() -> (w473:cluster{i32, i32}[][])
                    n332 = local read "BackGround"() -> (w477:picture)
                    n333 = local read "ShipMap"() -> (w476:u32[][])
                    n334 = DataSocket Open(10:T10."Read" ("mode"), 11:w469) -> (3:w467:refnum<k13>)  [unwired: 2 in, 1 out]
                    n335 = DataSocket Read(11:w467) -> (3:w466:refnum<k13>)  [unwired: 4 in, 6 out]
                    n336 = Bundle("BackGround"=w477, "ShipMap"=w476, "ShipOneArray"=w475, "ShipTwoArray"=w474, "ShipThreeArray"=w473, "ShipFourArray"=w472) -> (w471:T3)  [unwired: 1 in]
                    n337 = while {
                      tunnel: [w482] -> w470
                      tunnel: w471 -> [w479]
                      tunnel: w466 -> [w478]
                      stop <- w483 stop-if-true
                      n338 = DataSocket Read(9:1000 ("ms timeout (10000)"), 10:w479, 11:w478) -> (1:w480:bool, 2:w482:T3)  [unwired: 2 in, 5 out]
                      "timed out 2" <- w480
                      n339 = Not(x=w480) -> (.not. x?=w483:bool)
                    }
                    "InputFromEnermy 2" <- w470
                  }
                  frame True {
                    n340 = local read "URLSend"() -> (w485:string)
                    n341 = local read "ShipFourArray"() -> (w488:cluster{i32, i32}[][])
                    n342 = local read "ShipTwoArray"() -> (w490:cluster{i32, i32}[][])
                    n343 = local read "ShipOneArray"() -> (w491:cluster{i32, i32}[][])
                    n344 = local read "ShipThreeArray"() -> (w489:cluster{i32, i32}[][])
                    n345 = local read "BackGround"() -> (w493:picture)
                    n346 = local read "ShipMap"() -> (w492:u32[][])
                    n347 = DataSocket Open(10:T10."Write" ("mode"), 11:w485) -> (3:w484:refnum<k13>)  [unwired: 2 in, 1 out]
                    n348 = Bundle("BackGround"=w493, "ShipMap"=w492, "ShipOneArray"=w491, "ShipTwoArray"=w490, "ShipThreeArray"=w489, "ShipFourArray"=w488) -> (w487:T3)  [unwired: 1 in]
                    n349 = DataSocket Write(10:w487, 11:w484) -> ()  [unwired: 2 in, 3 out]
                  }
                }
              }
              frame #3 {
                n350 = local read "ClientFirst?"() -> (w494:bool)
                n351 = case shown="False" w494 {
                  frame False {
                    n352 = local read "InputFromEnermy"() -> (w496:T3)
                    n353 = Unbundle By Name(w496) -> ("BackGround"=w495:picture, "ShipMap"=w497:u32[][], "ShipOneArray"=w498:cluster{i32, i32}[][], "ShipTwoArray"=w499:cluster{i32, i32}[][], "ShipThreeArray"=w500:cluster{i32, i32}[][], "ShipFourArray"=w501:cluster{i32, i32}[][])
                    n354 = local write "ShipThreeArray"(w500) -> ()
                    n355 = local write "ShipOneArray"(w498) -> ()
                    n356 = local write "ShipTwoArray"(w499) -> ()
                    n357 = local write "ShipFourArray"(w501) -> ()
                    n358 = local write "ShipMap"(w497) -> ()
                    n359 = local write "PictureOut"(w495) -> ()
                  }
                  frame True {
                    n360 = local read "InputFromEnermy 2"() -> (w503:T3)
                    n361 = Unbundle By Name(w503) -> ("BackGround"=w502:picture, "ShipMap"=w504:u32[][], "ShipOneArray"=w505:cluster{i32, i32}[][], "ShipTwoArray"=w506:cluster{i32, i32}[][], "ShipThreeArray"=w507:cluster{i32, i32}[][], "ShipFourArray"=w508:cluster{i32, i32}[][])
                    n362 = local write "ShipThreeArray"(w507) -> ()
                    n363 = local write "ShipOneArray"(w505) -> ()
                    n364 = local write "ShipTwoArray"(w506) -> ()
                    n365 = local write "ShipFourArray"(w508) -> ()
                    n366 = local write "ShipMap"(w504) -> ()
                    n367 = local write "PictureOut"(w502) -> ()
                  }
                }
              }
            }
          }
        }
        n368 = local read "ClientFirst?"() -> (w393:bool)
        n369 = Select(t=T6."MyTurn", s=w393, f=T6."EnermyTurn") -> (s? t:f=w391:T6)
      }
      frame "MyTurn" {
        n370 = flat-sequence {
          tunnel: [w745] -> w510
          frame #0 {
            n371 = while {
              stop <- w513 stop-if-true
              n372 = local read "TimeToChangeTurn"() -> (w512:bool)
              n373 = case shown="False" w512 {
                frame False {
                  n374 = flat-sequence {
                    frame #0 {
                      n375 = while {
                        stop <- w514 stop-if-true
                        w518 = 20
                        w523 = 20
                        n376 = local read "MouseLocation"() -> (w526:T4)
                        n377 = Unbundle(w526) -> ("Horizontal"=w525:i32, "Vertical"=w524:i32)
                        n378 = Quotient & Remainder(x=w525, y=w523) -> (floor(x/y)=w520:i32)  [unwired: 1 out]
                        n379 = Quotient & Remainder(x=w524, y=w523) -> (floor(x/y)=w519:i32)  [unwired: 1 out]
                        n380 = Multiply(x=w520, y=w518) -> (x*y=w516:i32)
                        n381 = Multiply(x=w518, y=w519) -> (x*y=w517:i32)
                        n382 = local read "MouseButtonDown"() -> (w514:bool)
                        n383 = Bundle(w516, w517) -> (w522:cluster{i32, i32})  [unwired: 1 in]
                        n384 = Add(x=w522, y=cluster{i32, i32} {459, 111}) -> (x+y=w515:cluster{i32, i32})
                        n385 = property on="Boolean" class="Bool (strict)"("Position"=w515) -> ()  [unwired: 2 in, 2 out]
                      }
                    }
                    frame #1 {
                      w527 = FALSE
                      w535 = 20 ("y")
                      n386 = local read "MouseLocation"() -> (w538:T4)
                      n387 = local read "BattleShipFace"() -> (w539:bool[][])
                      n388 = Unbundle(w538) -> ("Horizontal"=w537:i32, "Vertical"=w536:i32)
                      n389 = Quotient & Remainder(x=w537, y=w535) -> (floor(x/y)=w531:i32)  [unwired: 1 out]
                      n390 = Quotient & Remainder(x=w536, y=w535) -> (floor(x/y)=w530:i32)  [unwired: 1 out]
                      n391 = Replace Array Subset(array=w539, new element=FALSE ("new element/subarray"), index (row)=w530, index (col)=w531) -> (w534:bool[][])
                      n392 = local write "BattleShipFace"(w534) -> ()
                      n393 = local read "ShipMap"() -> (w532:u32[][])
                      n394 = Bundle(w531, w530) -> (→"SendLocation":cluster{i32, i32})  [unwired: 1 in]
                      n395 = Index Array(array=w532, index (row)=w530, index (col)=w531) -> (element=→"HitIndex":u32)
                      n396 = local write "x .and. y? 3"(w527) -> ()
                      n397 = local write "x .and. y? 4"(w527) -> ()
                      n398 = local write "x .and. y? 2"(w527) -> ()
                      n399 = local write "x .and. y?"(w527) -> ()
                    }
                    frame #2 {
                      n400 = local read "HitIndex"() -> (w540:u32)
                      n401 = case shown="3" w540 {
                        frame 0, Default {
                        }
                        frame 1 {
                          n402 = local read "ShipOneArray"() -> (w541:cluster{i32, i32}[][])
                          n403 = for {
                            tunnel: w541 -> [w544] mode=indexing
                            i -> [w542]
                            stop <- w543 stop-if-true
                            n404 = for {
                              tunnel: w544 -> [w555] mode=indexing
                              tunnel: w542 -> [w547]
                              i -> [w546]
                              stop <- w545 stop-if-true
                              n405 = local read "SendLocation"() -> (w554:cluster{i32, i32})
                              n406 = Unbundle(w555) -> (w551:i32, w553:i32)
                              n407 = Unbundle(w554) -> (w552:i32, w550:i32)
                              n408 = Equal?(x=w552, y=w551) -> (x = y?=w548:bool)
                              n409 = Equal?(x=w550, y=w553) -> (x = y?=w549:bool)
                              n410 = And(x=w549, y=w548) -> (x .and. y?=w545:bool)
                              "x .and. y?" <- w545
                              n411 = case shown="True" w545 {
                                tunnel: w547 -> [_ w557]
                                tunnel: w546 -> [_ w556]
                                frame False {
                                }
                                frame True {
                                n412 = flat-sequence {
                                tunnel: w557 -> [w563]
                                tunnel: w556 -> [w562]
                                frame #0 {
                                n413 = local read "ShipOneArray"() -> (w564:cluster{i32, i32}[][])
                                n414 = Bundle(100, 100) -> (w559:cluster{i32, i32})  [unwired: 1 in]
                                n415 = Replace Array Subset(array=w564, new element=w559, index (row)=w563, index (col)=w562) -> (w558:cluster{i32, i32}[][])
                                n416 = local write "ShipOneArray"(w558) -> ()
                                }
                                frame #1 {
                                n417 = local read "ShipOneArray"() -> (w565:cluster{i32, i32}[][])
                                n418 = for {
                                tunnel: w565 -> [w568] mode=indexing
                                i -> [w566]
                                n419 = for {
                                shift-right: [w576] -> w567
                                shift-left: TRUE -> [w577]
                                tunnel: w568 -> [w583] mode=indexing
                                w580 = 100 ("y")
                                n420 = Unbundle(w583) -> (w582:i32, w581:i32)
                                n421 = Equal?(x=w582, y=w580) -> (x = y?=w579:bool)
                                n422 = Equal?(x=w580, y=w581) -> (x = y?=w578:bool)
                                n423 = Compound Arithmetic op=AND(w579, w578, w577) -> (w576:bool)
                                }
                                n424 = case shown="True" w567 {
                                tunnel: w566 -> [_ w574]
                                frame False {
                                }
                                frame True {
                                n425 = local read "ShipOneArray"() -> (w575:cluster{i32, i32}[][])
                                n426 = local read "HitIndex"() -> (w572:u32)
                                n427 = Delete From Array(array=w575, index (row)=w574) -> (array with subset deleted=w573:cluster{i32, i32}[][])  [unwired: 2 in, 1 out]
                                n428 = local write "ShipOneArray"(w573) -> ()
                                n429 = Add(x=w572, y=u32 4) -> (x+y=w570:u32)
                                n430 = local write "HitIndex"(w570) -> ()
                                }
                                }
                                }
                                }
                                }
                                }
                              }
                            }
                            n431 = local read "x .and. y?"() -> (w543:bool)
                          }
                        }
                        frame 2 {
                          n432 = local read "ShipTwoArray"() -> (w584:cluster{i32, i32}[][])
                          n433 = for {
                            tunnel: w584 -> [w587] mode=indexing
                            i -> [w585]
                            stop <- w586 stop-if-true
                            n434 = for {
                              tunnel: w587 -> [w598] mode=indexing
                              tunnel: w585 -> [w590]
                              i -> [w589]
                              stop <- w588 stop-if-true
                              n435 = local read "SendLocation"() -> (w597:cluster{i32, i32})
                              n436 = Unbundle(w598) -> (w594:i32, w596:i32)
                              n437 = Unbundle(w597) -> (w595:i32, w593:i32)
                              n438 = Equal?(x=w595, y=w594) -> (x = y?=w591:bool)
                              n439 = Equal?(x=w593, y=w596) -> (x = y?=w592:bool)
                              n440 = And(x=w592, y=w591) -> (x .and. y?=w588:bool)
                              "x .and. y? 2" <- w588
                              n441 = case shown="True" w588 {
                                tunnel: w590 -> [_ w600]
                                tunnel: w589 -> [_ w599]
                                frame False {
                                }
                                frame True {
                                n442 = flat-sequence {
                                tunnel: w600 -> [w606]
                                tunnel: w599 -> [w605]
                                frame #0 {
                                n443 = local read "ShipTwoArray"() -> (w607:cluster{i32, i32}[][])
                                n444 = Bundle(100, 100) -> (w602:cluster{i32, i32})  [unwired: 1 in]
                                n445 = Replace Array Subset(array=w607, new element=w602, index (row)=w606, index (col)=w605) -> (w601:cluster{i32, i32}[][])
                                n446 = local write "ShipTwoArray"(w601) -> ()
                                }
                                frame #1 {
                                n447 = local read "ShipTwoArray"() -> (w608:cluster{i32, i32}[][])
                                n448 = for {
                                tunnel: w608 -> [w611] mode=indexing
                                i -> [w609]
                                n449 = for {
                                shift-right: [w619] -> w610
                                shift-left: TRUE -> [w620]
                                tunnel: w611 -> [w626] mode=indexing
                                w623 = 100 ("y")
                                n450 = Unbundle(w626) -> (w625:i32, w624:i32)
                                n451 = Equal?(x=w625, y=w623) -> (x = y?=w622:bool)
                                n452 = Equal?(x=w623, y=w624) -> (x = y?=w621:bool)
                                n453 = Compound Arithmetic op=AND(w622, w621, w620) -> (w619:bool)
                                }
                                n454 = case shown="True" w610 {
                                tunnel: w609 -> [_ w617]
                                frame False {
                                }
                                frame True {
                                n455 = local read "ShipTwoArray"() -> (w618:cluster{i32, i32}[][])
                                n456 = local read "HitIndex"() -> (w615:u32)
                                n457 = Delete From Array(array=w618, index (row)=w617) -> (array with subset deleted=w616:cluster{i32, i32}[][])  [unwired: 2 in, 1 out]
                                n458 = local write "ShipTwoArray"(w616) -> ()
                                n459 = Add(x=w615, y=u32 4) -> (x+y=w613:u32)
                                n460 = local write "HitIndex"(w613) -> ()
                                }
                                }
                                }
                                }
                                }
                                }
                              }
                            }
                            n461 = local read "x .and. y? 2"() -> (w586:bool)
                          }
                        }
                        frame 3 {
                          n462 = local read "ShipThreeArray"() -> (w627:cluster{i32, i32}[][])
                          n463 = for {
                            tunnel: w627 -> [w630] mode=indexing
                            i -> [w628]
                            stop <- w629 stop-if-true
                            n464 = for {
                              tunnel: w630 -> [w641] mode=indexing
                              tunnel: w628 -> [w633]
                              i -> [w632]
                              stop <- w631 stop-if-true
                              n465 = local read "SendLocation"() -> (w640:cluster{i32, i32})
                              n466 = Unbundle(w640) -> (w638:i32, w636:i32)
                              n467 = Unbundle(w641) -> (w637:i32, w639:i32)
                              n468 = Equal?(x=w638, y=w637) -> (x = y?=w634:bool)
                              n469 = Equal?(x=w636, y=w639) -> (x = y?=w635:bool)
                              n470 = And(x=w635, y=w634) -> (x .and. y?=w631:bool)
                              "x .and. y? 3" <- w631
                              n471 = case shown="True" w631 {
                                tunnel: w633 -> [_ w643]
                                tunnel: w632 -> [_ w642]
                                frame False {
                                }
                                frame True {
                                n472 = flat-sequence {
                                tunnel: w643 -> [w649]
                                tunnel: w642 -> [w648]
                                frame #0 {
                                n473 = local read "ShipThreeArray"() -> (w650:cluster{i32, i32}[][])
                                n474 = Bundle(100, 100) -> (w645:cluster{i32, i32})  [unwired: 1 in]
                                n475 = Replace Array Subset(array=w650, new element=w645, index (row)=w649, index (col)=w648) -> (w644:cluster{i32, i32}[][])
                                n476 = local write "ShipThreeArray"(w644) -> ()
                                }
                                frame #1 {
                                n477 = local read "ShipThreeArray"() -> (w651:cluster{i32, i32}[][])
                                n478 = for {
                                tunnel: w651 -> [w654] mode=indexing
                                i -> [w652]
                                n479 = for {
                                shift-right: [w662] -> w653
                                shift-left: TRUE -> [w663]
                                tunnel: w654 -> [w669] mode=indexing
                                w666 = 100 ("y")
                                n480 = Unbundle(w669) -> (w668:i32, w667:i32)
                                n481 = Equal?(x=w668, y=w666) -> (x = y?=w665:bool)
                                n482 = Equal?(x=w666, y=w667) -> (x = y?=w664:bool)
                                n483 = Compound Arithmetic op=AND(w665, w664, w663) -> (w662:bool)
                                }
                                n484 = case shown="True" w653 {
                                tunnel: w652 -> [_ w660]
                                frame False {
                                }
                                frame True {
                                n485 = local read "ShipThreeArray"() -> (w661:cluster{i32, i32}[][])
                                n486 = local read "HitIndex"() -> (w658:u32)
                                n487 = Delete From Array(array=w661, index (row)=w660) -> (array with subset deleted=w659:cluster{i32, i32}[][])  [unwired: 2 in, 1 out]
                                n488 = local write "ShipThreeArray"(w659) -> ()
                                n489 = Add(x=w658, y=u32 4) -> (x+y=w656:u32)
                                n490 = local write "HitIndex"(w656) -> ()
                                }
                                }
                                }
                                }
                                }
                                }
                              }
                            }
                            n491 = local read "x .and. y? 3"() -> (w629:bool)
                          }
                        }
                        frame 4 {
                          n492 = local read "ShipFourArray"() -> (w670:cluster{i32, i32}[][])
                          n493 = for {
                            tunnel: w670 -> [w673] mode=indexing
                            i -> [w671]
                            stop <- w672 stop-if-true
                            n494 = for {
                              tunnel: w673 -> [w684] mode=indexing
                              tunnel: w671 -> [w676]
                              i -> [w675]
                              stop <- w674 stop-if-true
                              n495 = local read "SendLocation"() -> (w683:cluster{i32, i32})
                              n496 = Unbundle(w684) -> (w680:i32, w682:i32)
                              n497 = Unbundle(w683) -> (w681:i32, w679:i32)
                              n498 = Equal?(x=w681, y=w680) -> (x = y?=w677:bool)
                              n499 = Equal?(x=w679, y=w682) -> (x = y?=w678:bool)
                              n500 = And(x=w678, y=w677) -> (x .and. y?=w674:bool)
                              "x .and. y? 4" <- w674
                              n501 = case shown="True" w674 {
                                tunnel: w676 -> [_ w686]
                                tunnel: w675 -> [_ w685]
                                frame False {
                                }
                                frame True {
                                n502 = flat-sequence {
                                tunnel: w686 -> [w692]
                                tunnel: w685 -> [w691]
                                frame #0 {
                                n503 = local read "ShipFourArray"() -> (w693:cluster{i32, i32}[][])
                                n504 = Bundle(100, 100) -> (w688:cluster{i32, i32})  [unwired: 1 in]
                                n505 = Replace Array Subset(array=w693, new element=w688, index (row)=w692, index (col)=w691) -> (w687:cluster{i32, i32}[][])
                                n506 = local write "ShipFourArray"(w687) -> ()
                                }
                                frame #1 {
                                n507 = local read "ShipFourArray"() -> (w694:cluster{i32, i32}[][])
                                n508 = for {
                                tunnel: w694 -> [w697] mode=indexing
                                i -> [w695]
                                n509 = for {
                                shift-right: [w705] -> w696
                                shift-left: TRUE -> [w706]
                                tunnel: w697 -> [w712] mode=indexing
                                w709 = 100 ("y")
                                n510 = Unbundle(w712) -> (w711:i32, w710:i32)
                                n511 = Equal?(x=w711, y=w709) -> (x = y?=w708:bool)
                                n512 = Equal?(x=w709, y=w710) -> (x = y?=w707:bool)
                                n513 = Compound Arithmetic op=AND(w708, w707, w706) -> (w705:bool)
                                }
                                n514 = case shown="True" w696 {
                                tunnel: w695 -> [_ w703]
                                frame False {
                                }
                                frame True {
                                n515 = local read "ShipFourArray"() -> (w704:cluster{i32, i32}[][])
                                n516 = local read "HitIndex"() -> (w701:u32)
                                n517 = Delete From Array(array=w704, index (row)=w703) -> (array with subset deleted=w702:cluster{i32, i32}[][])  [unwired: 2 in, 1 out]
                                n518 = local write "ShipFourArray"(w702) -> ()
                                n519 = Add(x=w701, y=u32 4) -> (x+y=w699:u32)
                                n520 = local write "HitIndex"(w699) -> ()
                                }
                                }
                                }
                                }
                                }
                                }
                              }
                            }
                            n521 = local read "x .and. y? 4"() -> (w672:bool)
                          }
                        }
                      }
                    }
                    frame #3 {
                      n522 = local read "ShipThreeArray"() -> (w724:cluster{i32, i32}[][])
                      n523 = local read "ShipOneArray"() -> (w726:cluster{i32, i32}[][])
                      n524 = local read "ShipFourArray"() -> (w723:cluster{i32, i32}[][])
                      n525 = local read "ShipTwoArray"() -> (w725:cluster{i32, i32}[][])
                      n526 = local read "HitIndex"() -> (w717:u32)
                      n527 = local read "HitArray"() -> (w715:picture[])
                      n528 = Empty Array?(array=w726) -> (empty?=w722:bool)
                      n529 = Empty Array?(array=w723) -> (empty?=w719:bool)
                      n530 = Empty Array?(array=w724) -> (empty?=w720:bool)
                      n531 = Empty Array?(array=w725) -> (empty?=w721:bool)
                      n532 = Compound Arithmetic op=AND(w722, w721, w720, w719) -> (w718:bool)
                      n533 = Select(t=u32 9, s=w718, f=w717) -> (s? t:f=w714:u32)
                      n534 = Index Array(array=w715, index=w714) -> (element=w713:picture)
                      n535 = local write "HitIndex"(w714) -> ()
                      n536 = local write "HitPicture"(w713) -> ()
                    }
                    frame #4 {
                      n537 = local read "HitIndex"() -> (w727:u32)
                      n538 = case shown="9" w727 {
                        frame 0, Default {
                          n539 = local write "PlayMusic"(2 ("PlayMusic")) -> ()
                        }
                        frame 1..4 {
                          n540 = local write "PlayMusic"(3 ("PlayMusic")) -> ()
                        }
                        frame 5..8 {
                          n541 = local write "PlayMusic"(4 ("PlayMusic")) -> ()
                        }
                        frame 9 {
                          n542 = local write "PlayMusic"(5 ("PlayMusic")) -> ()
                        }
                      }
                    }
                    frame #5 {
                      n543 = local read "URLSend"() -> (w737:string)
                      n544 = DataSocket Open(10:T10."Write" ("mode"), 11:w737) -> (3:w732:refnum<k13>)  [unwired: 2 in, 1 out]
                      n545 = local read "SendLocation"() -> (w734:cluster{i32, i32})
                      n546 = local read "HitIndex"() -> (w735:u32)
                      n547 = Bundle("HitIndex"=w735, "SendLocation"=w734) -> (w733:T2)  [unwired: 1 in]
                      "SendFormat" <- w733
                      n548 = DataSocket Write(10:w733, 11:w732) -> ()  [unwired: 2 in, 3 out]
                    }
                    frame #6 {
                      n549 = local write "MouseButtonDown"(FALSE ("MouseButtonDown")) -> ()
                    }
                    frame #7 {
                      n550 = local read "HitIndex"() -> (w742:u32)
                      "HitIndex 4" <- w742
                      n551 = Equal?(x=w742, y=u32 9) -> (x = y?=w740:bool)
                      n552 = Equal To 0?(x=w742) -> (x = 0?=w743:bool)
                      n553 = Or(x=w743, y=w740) -> (x .or. y?=→"TimeToChangeTurn":bool)
                    }
                  }
                }
                frame True {
                }
              }
              n554 = local read "TimeToChangeTurn"() -> (w513:bool)
            }
          }
          frame #1 {
            n555 = local read "HitIndex"() -> (w747:u32)
            "HitIndex 3" <- w747
            n556 = Equal?(x=w747, y=u32 9) -> (x = y?=w748:bool)
            n557 = Select(t=T1."GameOver" ("Enum 2"), s=w748, f=T1."EnermyTurn" ("Enum 2")) -> (s? t:f=w745:T1)
          }
        }
        n558 = property on="BattleShipFace" class="Arr (strict)"("DisabledEnum"=T8."Enabled" ("Disabled")) -> ()  [unwired: 2 in, 2 out]
        n559 = local write "TimeToChangeTurn2"(FALSE ("MouseButtonDown")) -> ()
      }
      frame "EnermyTurn" {
        n560 = flat-sequence {
          tunnel: [w796] -> w751
          frame #0 {
            n561 = while {
              stop <- w755 stop-if-true
              n562 = local read "TimeToChangeTurn2"() -> (w754:bool)
              n563 = case shown="False" w754 {
                frame False {
                  n564 = flat-sequence {
                    frame #0 {
                      n565 = local read "URLReceive"() -> (w761:string)
                      n566 = DataSocket Open(10:T10."Read" ("mode"), 11:w761) -> (3:w757:refnum<k13>)  [unwired: 2 in, 1 out]
                      n567 = DataSocket Read(11:w757) -> (3:w756:refnum<k13>)  [unwired: 4 in, 6 out]
                      n568 = while {
                        tunnel: w756 -> [w767]
                        stop <- w763 stop-if-true
                        n569 = local read "SendFormat"() -> (w766:T2)
                        n570 = DataSocket Read(9:1000 ("ms timeout (10000)"), 10:w766, 11:w767) -> (1:w762:bool, 2:→"DataTemp":T2)  [unwired: 2 in, 5 out]
                        "timed out 3" <- w762
                        n571 = Not(x=w762) -> (.not. x?=w763:bool)
                      }
                      n572 = local read "Counter"() -> (w759:i32)
                      n573 = Increment(x=w759) -> (x+1=w758:i32)
                      n574 = local write "Counter"(w758) -> ()
                    }
                    frame #1 {
                      n575 = local read "DataTemp"() -> (w778:T2)
                      n576 = local read "HitArray"() -> (w780:picture[])
                      n577 = Unbundle(w778) -> ("HitIndex"=w770:u32, "SendLocation"=w782:cluster{i32, i32})
                      "HitIndex 2" <- w770
                      n578 = local read "BackGroundFace"() -> (w777:bool[][])
                      n579 = Unbundle(w782) -> (w776:i32, w775:i32)
                      n580 = Equal?(x=w770, y=u32 9) -> (x = y?=w773:bool)
                      n581 = Select(t=u32 10, s=w773, f=w770) -> (s? t:f=w771:u32)
                      n582 = Index Array(array=w780, index=w771) -> (element=w781:picture)
                      n583 = local read "Counter"() -> (w768:i32)
                      n584 = local write "HitPicture"(w781) -> ()
                      n585 = Replace Array Subset(array=w777, new element=TRUE ("new element/subarray"), index (row)=w775, index (col)=w776) -> (w783:bool[][])
                      n586 = Increment(x=w768) -> (x+1=w769:i32)
                      n587 = local write "BackGroundFace"(w783) -> ()
                      n588 = local write "Counter"(w769) -> ()
                    }
                    frame #2 {
                      n589 = local read "HitIndex 2"() -> (w790:u32)
                      n590 = local read "Counter"() -> (w785:i32)
                      n591 = Equal To 0?(x=w790) -> (x = 0?=w788:bool)
                      n592 = Equal?(x=w790, y=u32 9) -> (x = y?=w787:bool)
                      n593 = Or(x=w788, y=w787) -> (x .or. y?=→"TimeToChangeTurn2":bool)
                      n594 = Increment(x=w785) -> (x+1=w784:i32)
                      n595 = local write "Counter"(w784) -> ()
                    }
                    frame #3 {
                      n596 = local read "HitIndex 2"() -> (w791:u32)
                      n597 = case shown="9" w791 {
                        frame 0, Default {
                          n598 = local write "PlayMusic"(2 ("PlayMusic")) -> ()
                        }
                        frame 1..4 {
                          n599 = local write "PlayMusic"(3 ("PlayMusic")) -> ()
                        }
                        frame 5..8 {
                          n600 = local write "PlayMusic"(8 ("PlayMusic")) -> ()
                        }
                        frame 9 {
                          n601 = local write "PlayMusic"(6 ("PlayMusic")) -> ()
                        }
                      }
                    }
                  }
                }
                frame True {
                }
              }
              n602 = local read "TimeToChangeTurn2"() -> (w755:bool)
              "TimeToChangeTurn2 2" <- w755
            }
          }
          frame #1 {
            n603 = local read "HitIndex 2"() -> (w797:u32)
            n604 = Equal?(x=w797, y=u32 9) -> (x = y?=w799:bool)
            n605 = Select(t=T1."GameOver" ("Enum 2"), s=w799, f=T1."MyTurn" ("Enum 2")) -> (s? t:f=w796:T1)
          }
        }
        n606 = local write "MouseButtonDown"(FALSE ("MouseButtonDown")) -> ()
        n607 = local write "TimeToChangeTurn"(FALSE ("TimeToChangeTurn")) -> ()
        n608 = property on="BattleShipFace" class="Arr (strict)"("DisabledEnum"=T8."Disabled" ("Disabled")) -> ()  [unwired: 2 in, 2 out]
      }
      frame "GameOver" {
        n609 = local write "PlayMusic"(7 ("PlayMusic")) -> ()
      }
    }
    "Enum" <- w230
  }
  n610 = while {
    stop <- FALSE stop-if-true
    n611 = local read "PlayMusic"() -> (w805:i32)
    n612 = case shown="5" w805 {
      frame 0, Default {
      }
      frame 1 {
        n613 = local read "BasePath"() -> (w807:path)
        n614 = Build Path(base path=w807, name or relative path="Ready.wav") -> (appended path=w806:path)
        n615 = local write "PlayMusic"(0 ("PlayMusic")) -> ()
        n616 = call <vilib>:"Sound File Read Simple.vi"("path"=w806) -> ("data"=w810:waveform(dbl)[])  [unwired: 7 in, 3 out]
        n617 = call "Play Waveform2"("Data"=w810) -> ()  [unwired: 18 in, 1 out]
      }
      frame 2 {
        n618 = local read "BasePath"() -> (w812:path)
        n619 = Build Path(base path=w812, name or relative path="Miss.wav") -> (appended path=w811:path)
        n620 = local write "PlayMusic"(0 ("PlayMusic")) -> ()
        n621 = call <vilib>:"Sound File Read Simple.vi"("path"=w811) -> ("data"=w815:waveform(dbl)[])  [unwired: 7 in, 3 out]
        n622 = call "Play Waveform"("Data"=w815) -> ()  [unwired: 18 in, 1 out]
      }
      frame 3 {
        n623 = local read "BasePath"() -> (w817:path)
        n624 = Build Path(base path=w817, name or relative path="Hit.wav") -> (appended path=w816:path)
        n625 = local write "PlayMusic"(0 ("PlayMusic")) -> ()
        n626 = call <vilib>:"Sound File Read Simple.vi"("path"=w816) -> ("data"=w820:waveform(dbl)[])  [unwired: 7 in, 3 out]
        n627 = call "Play Waveform3"("Data"=w820) -> ()  [unwired: 18 in, 1 out]
      }
      frame 4 {
        n628 = local read "BasePath"() -> (w822:path)
        n629 = Build Path(base path=w822, name or relative path="Sunk.wav") -> (appended path=w821:path)
        n630 = local write "PlayMusic"(0 ("PlayMusic")) -> ()
        n631 = call <vilib>:"Sound File Read Simple.vi"("path"=w821) -> ("data"=w825:waveform(dbl)[])  [unwired: 7 in, 3 out]
        n632 = call "Play Waveform4"("Data"=w825) -> ()  [unwired: 18 in, 1 out]
      }
      frame 5 {
        n633 = local read "BasePath"() -> (w827:path)
        n634 = Build Path(base path=w827, name or relative path="Victory.wav") -> (appended path=w826:path)
        n635 = local write "PlayMusic"(0 ("PlayMusic")) -> ()
        n636 = call <vilib>:"Sound File Read Simple.vi"("path"=w826) -> ("data"=w830:waveform(dbl)[])  [unwired: 7 in, 3 out]
        n637 = call "Play Waveform5"("Data"=w830) -> ()  [unwired: 18 in, 1 out]
      }
      frame 6 {
        n638 = local read "BasePath"() -> (w832:path)
        n639 = Build Path(base path=w832, name or relative path="Defeat.wav") -> (appended path=w831:path)
        n640 = local write "PlayMusic"(0 ("PlayMusic")) -> ()
        n641 = call <vilib>:"Sound File Read Simple.vi"("path"=w831) -> ("data"=w835:waveform(dbl)[])  [unwired: 7 in, 3 out]
        n642 = call "Play Waveform6"("Data"=w835) -> ()  [unwired: 18 in, 1 out]
      }
      frame 7 {
        n643 = local read "BasePath"() -> (w837:path)
        n644 = Build Path(base path=w837, name or relative path="The_End.wav") -> (appended path=w836:path)
        n645 = local write "PlayMusic"(0 ("PlayMusic")) -> ()
        n646 = call <vilib>:"Sound File Read Simple.vi"("path"=w836) -> ("data"=w840:waveform(dbl)[])  [unwired: 7 in, 3 out]
        n647 = call "Play Waveform7"("Data"=w840) -> ()  [unwired: 18 in, 1 out]
      }
      frame 8 {
        n648 = local read "BasePath"() -> (w842:path)
        n649 = Build Path(base path=w842, name or relative path="No.wav") -> (appended path=w841:path)
        n650 = local write "PlayMusic"(0 ("PlayMusic")) -> ()
        n651 = call <vilib>:"Sound File Read Simple.vi"("path"=w841) -> ("data"=w845:waveform(dbl)[])  [unwired: 7 in, 3 out]
        n652 = call "Play Waveform8"("Data"=w845) -> ()  [unwired: 18 in, 1 out]
      }
    }
  }
  n653 = while {
    stop <- FALSE stop-if-true
    n654 = event shown="[1] \"Pane\": Mouse Move" {
      selector: _ -> [_ _ _]
      dyn-events: _ -> [_ _ _]
      timeout: _ -> [_ _ _]
      event Timeout {
        n655 = event-data() -> ()  [unwired: 1 in, 3 out]
      }
      event Mouse Move {
        n656 = event-data() -> ("Coords"=w849:T4)  [unwired: 1 in, 4 out]
        n657 = Subtract(x=w849, y=cluster{i32, i32} {459, 111}) -> (x-y=→"MouseLocation":T4)
      }
      event Mouse Down {
        w853 = 0 ("upper limit")
        w854 = 300 ("upper limit")
        n658 = event-data() -> ()  [unwired: 1 in, 8 out]
        n659 = local read "MouseLocation"() -> (w857:T4)
        n660 = Unbundle By Name(w857) -> ("Horizontal"=w856:i32, "Vertical"=w855:i32)
        n661 = In Range and Coerce(upper limit=w854, x=w856, lower limit=w853) -> (In Range?=w852:bool)  [unwired: 1 out]
        n662 = In Range and Coerce(upper limit=w854, x=w855, lower limit=w853) -> (In Range?=w851:bool)  [unwired: 1 out]
        n663 = And(x=w852, y=w851) -> (x .and. y?=w850:bool)
        n664 = local write "MouseButtonDown"(w850) -> ()
      }
    }
  }
  n665 = Current VI's Path() -> (path=w2:path)
  "path" <- w2
  n666 = Strip Path(path=w2) -> (stripped path=→"BasePath":path)  [unwired: 1 out]
  n667 = Initialize Array(cluster{i32, i32} {0, 0}, 0 ("dimension size")) -> (→"InitArray":cluster{i32, i32}[])
